vi "Telegram2Values.vi"(10 "index":i32, 11 "Value":string[](array[string])) -> (1 "Numeric 2":u16, 2 "Numeric 3":u16, 3 "Numeric 4":u16, 4 "Numeric":u16)   [LabVIEW 2012]
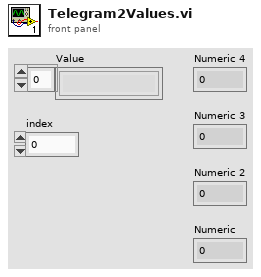
[diagram p1: front panel]
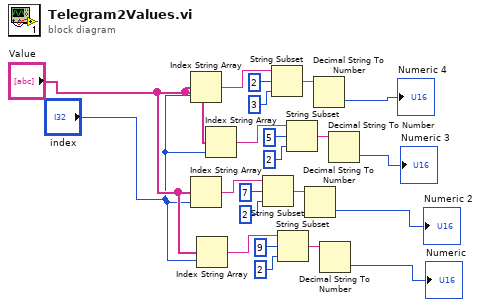
[diagram p0: block diagram]
diagram:
  n1 = Index String Array(1:"index", 2:"Value") -> (0:w4:string)  [unwired: 1 in]
  n2 = Index String Array(1:"index", 2:"Value") -> (0:w14:string)  [unwired: 1 in]
  n3 = Index String Array(1:"index", 2:"Value") -> (0:w18:string)  [unwired: 1 in]
  n4 = Index String Array(1:"index", 2:"Value") -> (0:w9:string)  [unwired: 1 in]
  n5 = String Subset(string=w14, offset (0)=7, length (rest)=2 ("length (rest)")) -> (substring=w13:string)
  n6 = String Subset(string=w4, offset (0)=2, length (rest)=3 ("length (rest)")) -> (substring=w3:string)
  n7 = String Subset(string=w18, offset (0)=9, length (rest)=2 ("length (rest)")) -> (substring=w17:string)
  n8 = String Subset(string=w9, offset (0)=5, length (rest)=2 ("length (rest)")) -> (substring=w8:string)
  n9 = Decimal String To Number(string=w13) -> (number=→"Numeric 2":i32)  [unwired: 2 in, 1 out]
  n10 = Decimal String To Number(string=w3) -> (number=→"Numeric 4":i32)  [unwired: 2 in, 1 out]
  n11 = Decimal String To Number(string=w17) -> (number=→"Numeric":i32)  [unwired: 2 in, 1 out]
  n12 = Decimal String To Number(string=w8) -> (number=→"Numeric 3":i32)  [unwired: 2 in, 1 out]
